vi "Sort Frames.vi"(8 "error in (no error)":errorcluster, 10 "Frames":refnum<k21>[](array[refnum]), 11 "CAN in":refnum<class "XNET_BS120x.lvclass">) -> (0 "error out":errorcluster, 3 "CAN out":refnum<class "XNET_BS120x.lvclass">)   [LabVIEW 2021, in "BS120x Driver.lvlib" / "XNET_BS120x.lvclass"]
uses:
  XNET_BS120x.lvclass
  XNET_BS120x.lvclass/XNET_BS120x.ctl
  <resource>/objmgr/xnet.rc
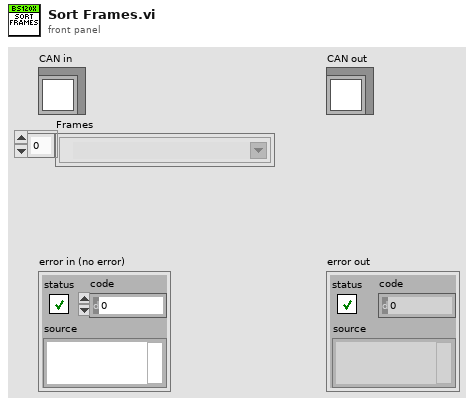
[diagram p1: front panel]
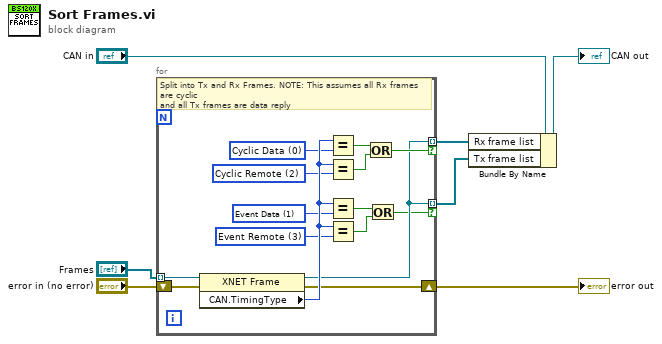
[diagram p0: block diagram]
diagram:
  n1 = for {
    tunnel: "Frames" -> [w22] mode=indexing
    shift-right: [w14] -> w4
    shift-left: "error in (no error)" -> [w21]
    tunnel: [w13] -> w6 mode=indexing if=w15
    tunnel: [w13] -> w5 mode=indexing if=w12
    w8 = u32 3 items=["Cyclic Data", "Event Data", "Cyclic Remote", "Event Remote", "Cyclic/Event"] ("CAN:Timing Type")
    w9 = u32 1 items=["Cyclic Data", "Event Data", "Cyclic Remote", "Event Remote", "Cyclic/Event"] ("CAN:Timing Type")
    w10 = u32 2 items=["Cyclic Data", "Event Data", "Cyclic Remote", "Event Remote", "Cyclic/Event"] ("CAN:Timing Type")
    w11 = u32 0 items=["Cyclic Data", "Event Data", "Cyclic Remote", "Event Remote", "Cyclic/Event"] ("CAN:Timing Type")
    # "Split into Tx and Rx Frames. NOTE: This assumes all Rx frames are cyclic \nand all Tx frames are data reply"
    n2 = property class="XNET Frame"(reference=w22, error in=w21) -> (reference out=w13:refnum<k21>, error out=w14:errorcluster, "CAN.TimingType"=w20:u32)
    n3 = Equal?(x=w20, y=w11) -> (x = y?=w19:bool)
    n4 = Equal?(x=w20, y=w10) -> (x = y?=w16:bool)
    n5 = Equal?(x=w20, y=w9) -> (x = y?=w18:bool)
    n6 = Equal?(x=w20, y=w8) -> (x = y?=w17:bool)
    n7 = Or(x=w19, y=w16) -> (x .or. y?=w15:bool)
    n8 = Or(x=w18, y=w17) -> (x .or. y?=w12:bool)
  }
  "error out" <- w4
  n9 = Bundle By Name(cluster="CAN in", "Rx frame list"=w6, "Tx frame list"=w5) -> (→"CAN out":refnum<class "XNET_BS120x.lvclass">)
